vi "Tone Frequency to Measurement Duration.vi"(7 "frequencies and measurement durations":cluster{"frequencies":dbl[], "durations":dbl[]}={"frequencies"=[0.0, 10.0, 20.0, 40.0, 80.0, 200.0], "durations"=[10.0, 2.0, 1.0, 0.5, 0.2, 0.1]}, 11 "tone frequency":dbl=1000.0) -> (3 "measurement duration":dbl)   [LabVIEW 2025, in "Tone Measurements.lvlib" / "Tone Measurements.lvclass"]
uses:
  Tone Measurements.lvclass
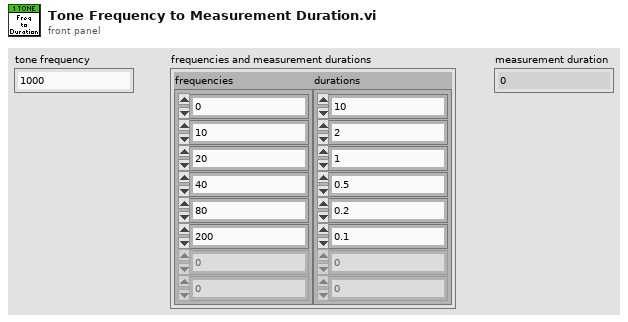
[diagram p1: front panel]
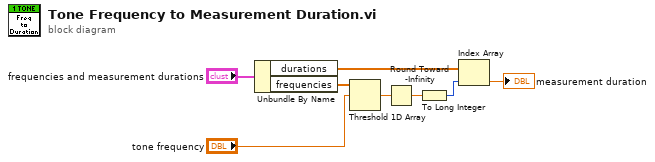
[diagram p0: block diagram]
diagram:
  n1 = Unbundle By Name("frequencies and measurement durations") -> ("durations"=w4:dbl[], "frequencies"=w5:dbl[])
  n2 = Threshold 1D Array(2:"tone frequency", 3:w5) -> (0:w7:dbl)  [unwired: 1 in]
  n3 = Round Toward -Infinity(1:w7) -> (0:w3:dbl)
  n4 = To Long Integer(number=w3) -> (32bit integer=w2:i32)
  n5 = Index Array(array=w4, index=w2) -> (element=→"measurement duration":dbl)
